vi "LVOS Public Repository.vi"() -> ()   [LabVIEW 2013]
uses:
  <vilib>/Utility/config.llb/Read Key (String).vi
  <vilib>/regexp/Match Regular Expression.xnode
  <vilib>/Utility/config.llb/NI_LVConfig.lvlib
panel:
  in  "LabVIEW Version":string="13.0"
  out "Version Matched":string[](array[string])
  out "Comparison":string[](array[string])
  out "file or folder exists? 2":bool
  out "file or folder exists?":bool
  in  "Repository Folder Location":path=path "C:/Users/Administrator/OneDrive/_DESIM/Package Repository"
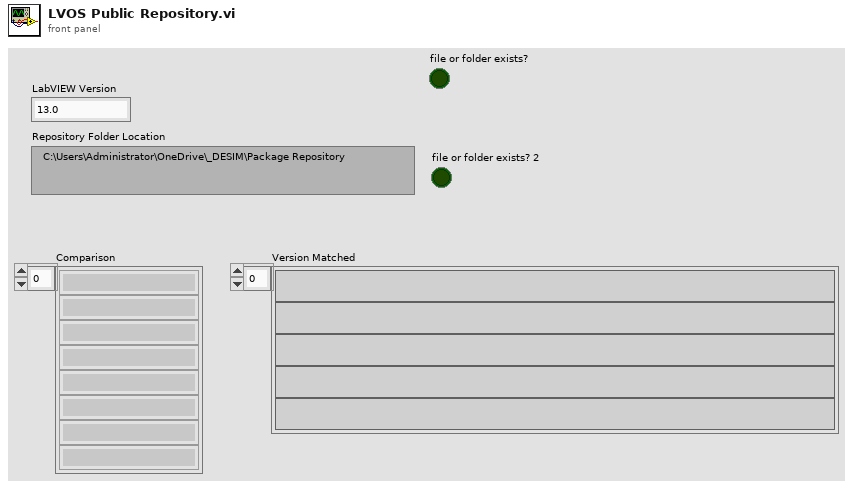
[diagram p1: front panel]
types:
  T1 = typedef "NI_LVConfig.lvlib/Config Data RefNum.ctl" = refnum<k1>
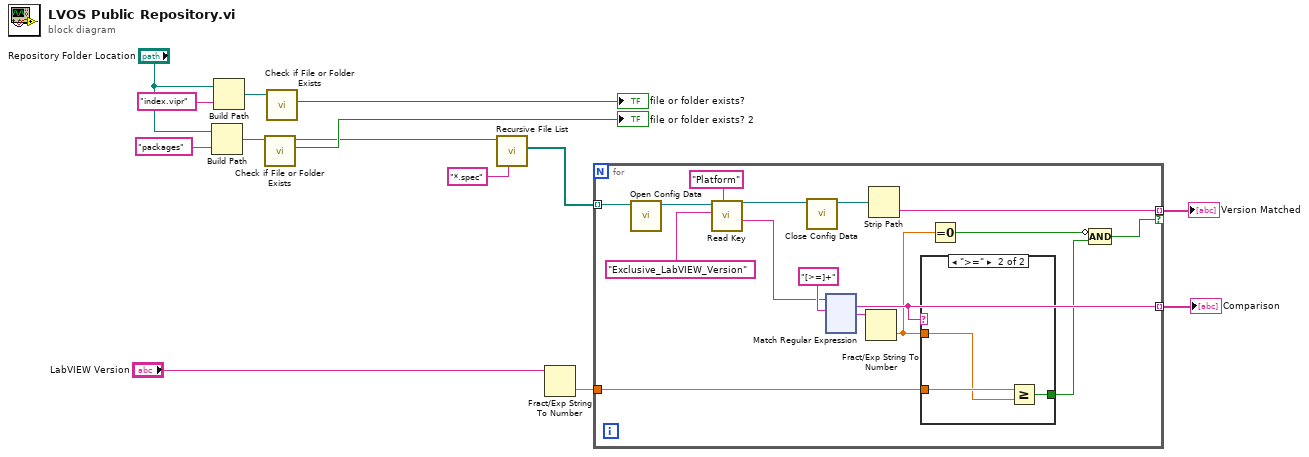
[diagram p0: block diagram]
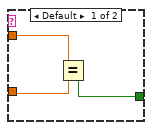
[diagram p2: hidden frame]
diagram:
  n1 = Build Path(base path="Repository Folder Location", name or relative path="packages") -> (appended path=w10:path)
  n2 = Build Path(base path="Repository Folder Location", name or relative path="index.vipr") -> (appended path=w11:path)
  n3 = call <vilib>:"Check if File or Folder Exists.vi"("path"=w10) -> ("file or folder exists?"=→"file or folder exists? 2":bool, "dup path"=w7:path)  [unwired: 8 in, 1 out]
  n4 = call <vilib>:"Check if File or Folder Exists.vi"("path"=w11) -> ("file or folder exists?"=→"file or folder exists?":bool)  [unwired: 8 in, 2 out]
  n5 = call <vilib>:"Recursive File List.vi"("pattern"="*.spec", "Folder Path"=w7) -> ("All Files in Dir"=w5:path[])  [unwired: 5 in, 4 out]
  n6 = Fract/Exp String To Number(string="LabVIEW Version") -> (number=w2:dbl)  [unwired: 3 in, 1 out]
  n7 = for {
    tunnel: w5 -> [w30] mode=indexing
    tunnel: [w21] -> w4 mode=indexing
    tunnel: w2 -> [w22]
    tunnel: [w15] -> w1 mode=indexing if=w18
    n8 = call <vilib>:"Open Config Data.vi"("configuration file path"=w30) -> ("refnum"=w29:T1)  [unwired: 8 in, 2 out]
    n9 = call-poly <vilib>:"Read Key.vi"("section"="Platform" ("pattern"), "key"="Exclusive_LabVIEW_Version" ("pattern"), "refnum"=w29) -> ("value"=w23:string, "refnum out"=w26:T1)  [unwired: 5 in, 2 out]
    n10 = call <vilib>:"Close Config Data.vi"("refnum"=w26) -> ("file path"=w16:path)  [unwired: 9 in, 1 out]
    n11 = xnode "Match Regular Expression"("input string"=w23, "regular expression"="[>=]+") -> ("whole match"=w21:string, "after match"=w24:string)  [unwired: 4 in, 3 out]
    n12 = Fract/Exp String To Number(string=w24) -> (number=w20:dbl)  [unwired: 3 in, 1 out]
    n13 = Strip Path(path=w16) -> (name=w15:string)  [unwired: 1 out]
    n14 = case shown="\">=\"" w21 {
      tunnel: w22 -> [w32 w36]
      tunnel: w20 -> [w33 w35]
      tunnel: [w31 w34] -> w17
      frame Default {
        n15 = Equal?(x=w33, y=w32) -> (x = y?=w31:bool)
      }
      frame ">=" {
        n16 = Greater Or Equal?(x=w36, y=w35) -> (x >= y?=w34:bool)
      }
    }
    n17 = Equal To 0?(x=w20) -> (x = 0?=w19:bool)
    n18 = Compound Arithmetic op=AND(invert w19, w17) -> (w18:bool)
  }
  "Comparison" <- w4
  "Version Matched" <- w1
